vi "OldClimbGlobal.vi"() -> ()   [LabVIEW 2023]
panel:
  out "ClimbSensorPoseLeft":dbl
  out "ClimbSensorPoseRight":dbl
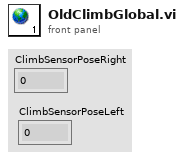
[diagram p1: front panel]
diagram:
